vi "Event Nested Teardown.vi"(11 "Base Queue jettl in":refnum<class "Base Queue jettl.lvclass">) -> (3 "Base Queue jettl out":refnum<class "Base Queue jettl.lvclass">)   [LabVIEW 2021, in "jettl.lvlib" / "Base Queue jettl.lvlib" / "Base Queue jettl.lvclass"]
uses:
  Base Queue jettl.lvclass
  Teardown/Teardown Msg Strategy/Teardown Msg Strategy.lvclass
  C:/git/jettl/src/jettl/Msg Strategy/Msg Strategy.lvclass
  Base Queue jettl.lvclass/Base Queue jettl.ctl
  Teardown/Teardown.lvlib
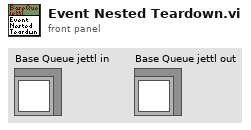
[diagram p1: front panel]
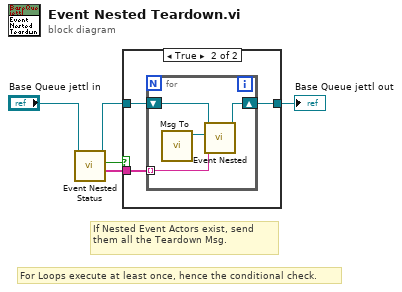
[diagram p0: block diagram]
diagram:
  # "If Nested Event Actors exist, send them all the Teardown Msg."
  # "For Loops execute at least once, hence the conditional check."
  n1 = call-dynamic "Event Nested Status.vi"("Base Queue jettl in"="Base Queue jettl in") -> ("Event Nested Aliases"=w4:string[], "Any Exist?"=w5:bool, "Base Queue jettl out"=w1:refnum<class "Base Queue jettl.lvclass">)  [unwired: 7 in, 1 out]
  n2 = case shown="True" w5 {
    tunnel: [w6 w9] -> w3
    tunnel: w1 -> [w6 w8]
    tunnel: w4 -> [_ w7]
    frame False {
    }
    frame True {
      n3 = for {
        tunnel: w7 -> [w11] mode=indexing
        shift-right: [w12] -> w9
        shift-left: w8 -> [w13]
        n4 = call "Msg To.vi"() -> ("Teardown Msg Strategy out"=w10:refnum<class "Teardown Msg Strategy.lvclass">)  [unwired: 11 in]
        n5 = call-dynamic "Event Nested.vi"("Alias"=w11, "Msg Strategy"=w10, "Base Queue jettl in"=w13) -> ("Base Queue jettl out"=w12:refnum<class "Base Queue jettl.lvclass">)  [unwired: 8 in]
      }
    }
  }
  "Base Queue jettl out" <- w3
